vi "Prepend Name if Modified.vi"(9 "Modified?":bool, 11 "VI Name":string) -> (3 "VI Name out":string)   [LabVIEW 2020, in "VI Properties Editor.lvlib"]
doc: "Prepends text to <B>VI Name in</B> based on <B>Modified?</B>."
uses:
  VI Properties Editor.lvlib
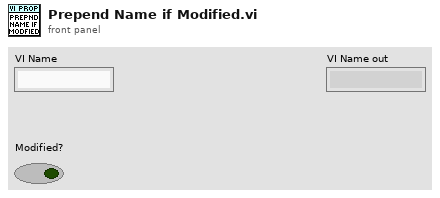
[diagram p1: front panel]
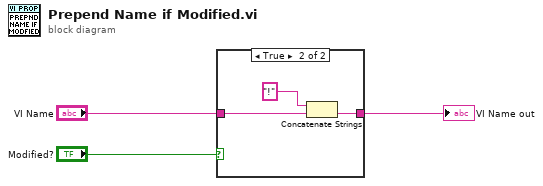
[diagram p0: block diagram]
diagram:
  n1 = case shown="True" "Modified?" {
    tunnel: [w4 w7] -> w1
    tunnel: "VI Name" -> [w4 w6]
    frame False {
    }
    frame True {
      n2 = Concatenate Strings("!" ("format string"), w6) -> (w7:string)
    }
  }
  "VI Name out" <- w1
